vi "_Save Users to File.vi"(8 "Error in":errorcluster caption="Error in (no error)", 11 "Array":T1[](array[typedef])) -> (0 "Error out":errorcluster)   [LabVIEW 2020, in "Login-UI.lvlib" / "PwdMgr.lvclass"]
uses:
  PwdMgr.lvclass
  _Typedef/User-Info.ctl
  _Typedef/User-Role.ctl
  4703436d-49e6-4ed7-825b-d682e24a79d8.vi
  <userlib>/NEVSTOP-Programming-Palette/Configuration/ClusterCfgTable/Flatten Cluster To CfgTable(with DataName).vi
  PwdMgr.lvclass/PwdMgr.ctl
  <userlib>/NEVSTOP-Programming-Palette/Configuration/Ini/ini_configuration_nevstop.lvlib
  <vilib>/NI/Tools/String/Tools_String.lvlib
  <userlib>/_NEVSTOP/Communicable State Machine(CSM)/Communicable State Machine.lvlib
  Login-UI.lvlib
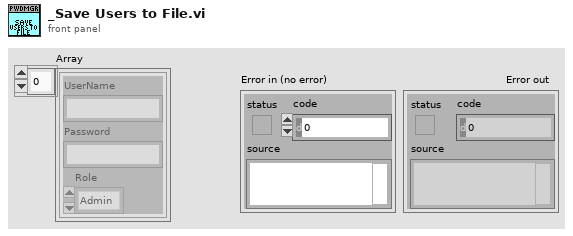
[diagram p1: front panel]
types:
  T1 = typedef "Login-UI.lvlib/User-Info.ctl" = cluster{"UserName":string, "Password":string, "Role":T2}
  T2 = typedef "Login-UI.lvlib/User-Role.ctl" = enum16{"INVALID", "Operator", "Engineer", "Admin", "Anonymous"}
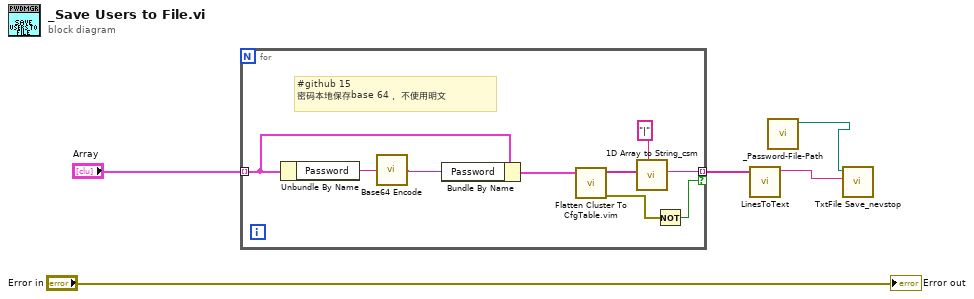
[diagram p0: block diagram]
diagram:
  n1 = for {
    tunnel: [w11] -> w3 mode=indexing if=w12
    tunnel: "Array" -> [w9] mode=indexing
    # "#github 15\n密码本地保存base 64， 不使用明文"
    n2 = Unbundle By Name(w9) -> ("Password"=w7:string)
    n3 = call <vilib>:"Base64 Encode.vi"("normal string"=w7) -> ("base64 string"=w6:string)  [unwired: 1 in]
    n4 = Bundle By Name(cluster=w9, "Password"=w6) -> (w8:T1)
    n5 = call "Flatten Cluster To CfgTable.vim"("Cluster Configuration Typedef"=w8) -> ("error out"=w13:errorcluster, "CfgTable Row"=w14:string[])  [unwired: 8 in, 1 out]
    n6 = call <userlib>:"1D Array to String_csm.vi"("delimiter (Tab)"="|", "Array of Strings"=w14) -> ("delimited string"=w11:string)  [unwired: 9 in]
    n7 = Not(x=w13) -> (.not. x?=w12:bool)
  }
  n8 = call <userlib>:"LinesToText.vi"("Lines"=w3) -> ("string"=w1:string)  [unwired: 9 in, 1 out]
  n9 = call "_Password-File-Path.vi"() -> ("Matched Config File"=w2:path)  [unwired: 11 in]
  n10 = call <userlib>:"TxtFile Save_nevstop.vi"("text"=w1, "Path"=w2) -> ()  [unwired: 9 in, 1 out]
  "Error out" <- "Error in"
